vi "set_disabled_state.vi"(8 "error in":errorcluster, 10 "status in":T1(ring)=enum."Disabled and Grayed Out", 11 "control references":refnum<vi>[](array[refnum])) -> (0 "error out":errorcluster)   [LabVIEW 2011]
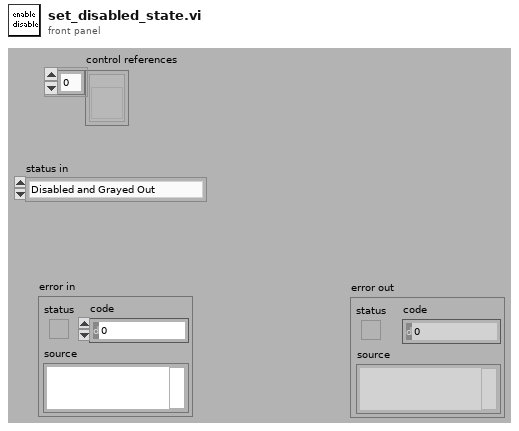
[diagram p1: front panel]
types:
  T1 = enum8{"Enabled", "Disabled", "Disabled and Grayed Out"}
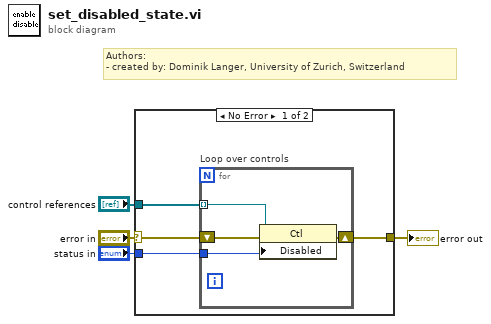
[diagram p0: block diagram]
diagram:
  # "Authors: \n- created by: Dominik Langer, University of Zurich, Switzerland"
  n1 = case shown="No Error" "error in" {
    selector: "error in" -> [w8 w13]
    tunnel: [w6 w13] -> w3
    tunnel: "control references" -> [w7 _]
    tunnel: "status in" -> [w5 _]
    frame No Error {
      n2 = for "Loop over controls" {
        shift-right: [w10] -> w6
        shift-left: w8 -> [w12]
        tunnel: w7 -> [w11] mode=indexing
        tunnel: w5 -> [w9]
        n3 = property class="Ctl"(reference=w11, error in=w12, "Disabled"=w9) -> (error out=w10:errorcluster)  [unwired: 1 out]
      }
    }
    frame Error {
    }
  }
  "error out" <- w3
